vi "PMX_ReadParameterSetNumber.vi"(8 "Error in":errorcluster, 11 "Device":refnum<k24>) -> (0 "Error out":errorcluster, 2 "CurrentParameterSetNumber":i32, 3 "Device":refnum<k24>)   [LabVIEW 2016]
doc: "Reads the currently loaded parameter set number (0,1,2,3...).\n\nDevice: PMX device on whicht to read the currently loaded parameter set number\nCurrentParametersetNumber: Currently loaded parameter set number (0,1,2,3,..)"
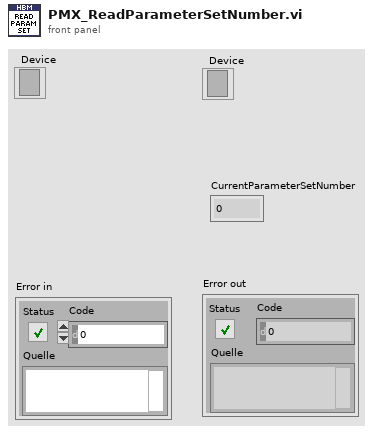
[diagram p1: front panel]
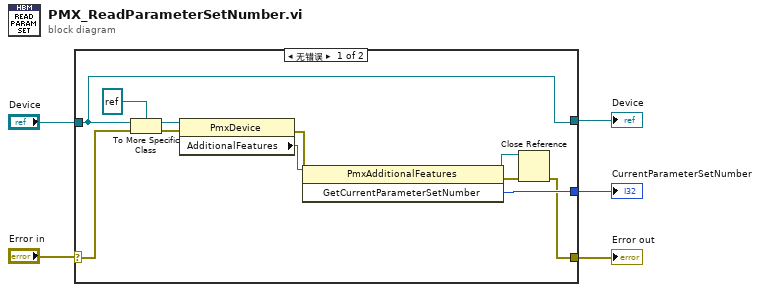
[diagram p0: block diagram]
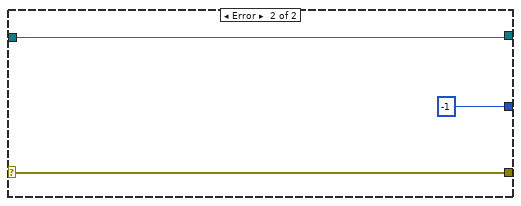
[diagram p2: hidden frame]
diagram:
  n1 = case shown="无错误" "Error in" {
    selector: "Error in" -> [w11 w19]
    tunnel: [w7 w19] -> w3
    tunnel: "Device" -> [w6 w18]
    tunnel: [w12 -1 ("GetCurrentParameterSetNumber")] -> w1
    tunnel: [w6 w18] -> w2
    frame No Error {
      n2 = To More Specific Class(target class=refnum<k24> refnum ("Zielklasse"), reference=w6, error in=w11) -> (specific class reference=w16:refnum<k24>, error out=w13:errorcluster)
      n3 = property on="Eigenschaftsknoten" class="PmxDevice"(reference=w16, error in=w13) -> (error out=w14:errorcluster, "AdditionalFeatures"=w15:refnum<k24>)  [unwired: 1 out]
      n4 = invoke on="Methodenknoten" class="PmxAdditionalFeatures" method="GetCurrentParameterSetNumber"(reference=w15, error in=w14) -> (reference out=w8:refnum<k24>, error out=w9:errorcluster, "GetCurrentParameterSetNumber"=w12:i32)  [unwired: 1 in]
      n5 = Close Reference(reference=w8, error in (no error)=w9) -> (error out=w7:errorcluster)
    }
    frame Error {
    }
  }
  "Error out" <- w3
  "Device" <- w2
  "CurrentParameterSetNumber" <- w1
